vi "test - MessageReponseNoError.vi"(8 "error in (no error)":errorcluster, 11 "TestCase in":refnum<class "testcase-SyncMessage.lvclass">) -> (0 "error out":errorcluster, 3 "TestCase out":refnum<class "testcase-SyncMessage.lvclass">)   [LabVIEW 2017, in "testcase-SyncMessage.lvclass"]
uses:
  testcase-SyncMessage.lvclass
  5ae9339b-24d8-490e-a9d6-72eb2a7b92ce.vi
  <vilib>/addons/_JKI Toolkits/VI Tester/TestCase.llb/TestCase.lvclass
  src/user.lib/_NEVSTOP/Communicable State Machine(CSM)/Communicable State Machine.lvlib
  C:/Program Files (x86)/National Instruments/LabVIEW 2017/vi.lib/addons/_JKI Toolkits/VI Tester/TestCase.llb/TestCase.lvclass
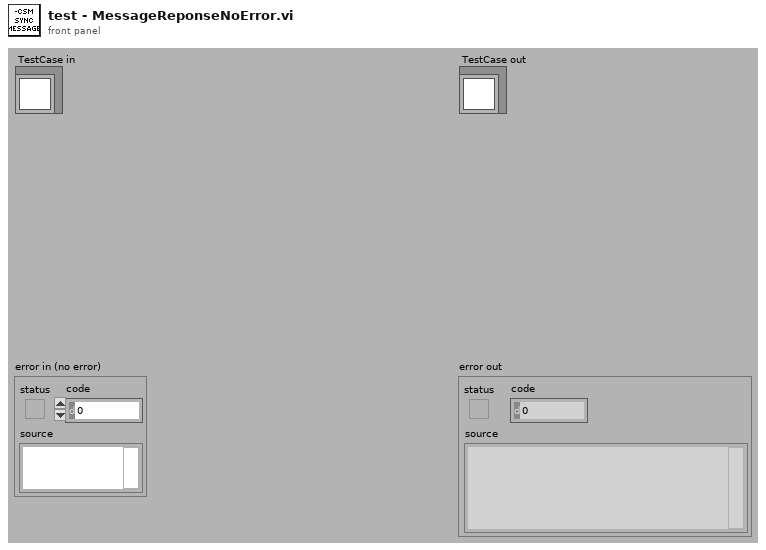
[diagram p1: front panel]
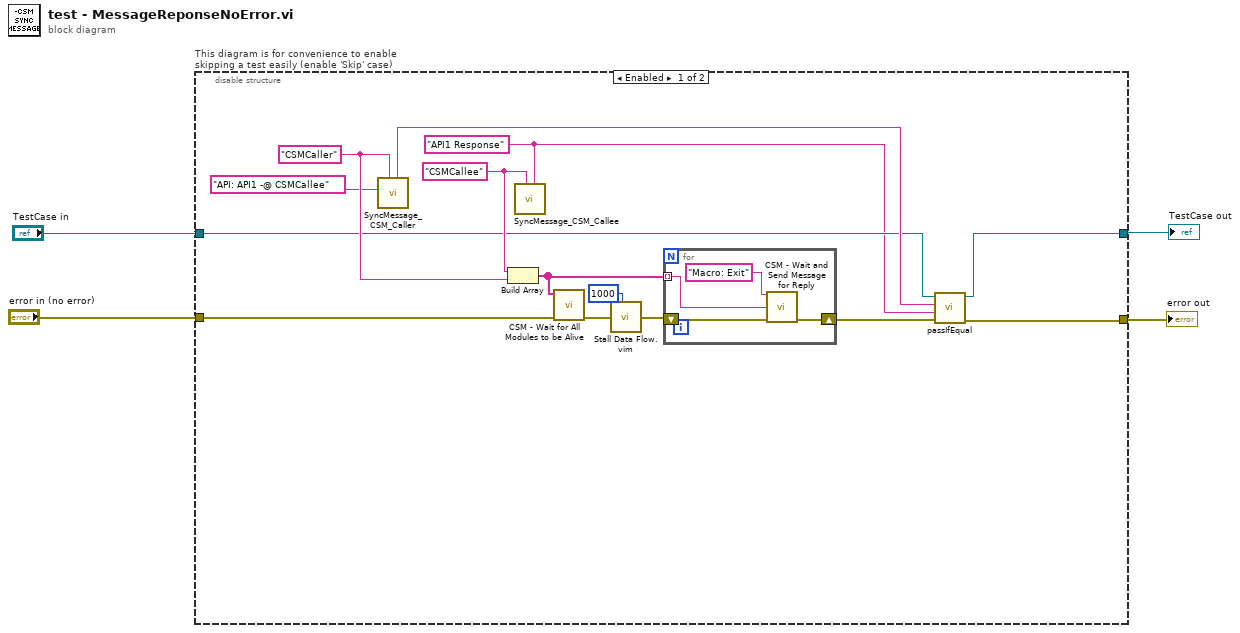
[diagram p0: block diagram]
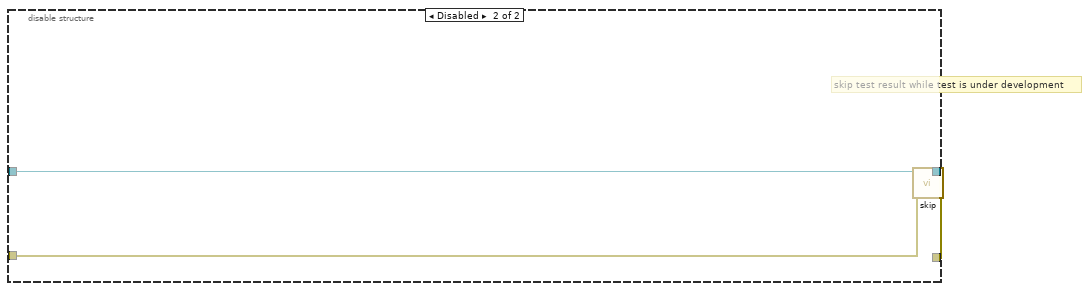
[diagram p2: hidden frame]
diagram:
  n1 = disable-structure "This diagram is for convenience to enable skipping a test easily (enable 'Skip' case)" shown="Enabled" {
    disable-tunnel: "TestCase in" -> [w7 w26]
    disable-tunnel: [w8 w24] -> w2
    disable-tunnel: [w9 w25] -> w1
    disable-tunnel: "error in (no error)" -> [w18 w23]
    frame Enabled {
      w6 = "API1 Response" ("API response in")
      w16 = "CSMCallee" ("Name (\"\" to Use UUID)")
      w17 = "CSMCaller" ("Name (\"\" to Use UUID)")
      n2 = call "SyncMessage_CSM_Caller.vi"("Name (\"\" to Use UUID)"=w17, "Intermodule Message in"="API: API1 -@ CSMCallee") -> ("API Response out"=w15:string)  [unwired: 9 in]
      n3 = Build Array(w16, w17) -> (w14:string[])
      n4 = call "SyncMessage_CSM_Callee.vi"("API response in"=w6, "Name (\"\" to Use UUID)"=w16) -> ()  [unwired: 10 in]
      n5 = call "CSM - Wait for All Modules to be Alive.vi"("Error In"=w18, "CSM Names"=w14) -> ("error out"=w13:errorcluster)  [unwired: 7 in, 2 out]
      n6 = call "Stall Data Flow.vim"("value in"=w13, "milliseconds to wait"=u32 1000) -> ("value out"=w12:errorcluster)  [unwired: 1 out]
      n7 = for {
        shift-right: [w20] -> w10
        shift-left: w12 -> [w21]
        tunnel: w14 -> [w19] mode=indexing
        n8 = call "CSM - Wait and Send Message for Reply.vi"("State"="Macro: Exit", "Target Module"=w19, "Error In (No Error)"=w21) -> ("error out"=w20:errorcluster)  [unwired: 10 in, 2 out]
      }
      n9 = call-dynamic "passIfEqual.vi"("error in (no error)"=w10, "y"=w6, "x"=w15, "TestCase in"=w7) -> ("error out"=w9:errorcluster, "TestCase out"=w8:refnum<class "testcase-SyncMessage.lvclass">)  [unwired: 6 in]
    }
    frame Disabled {
      # "skip test result while test is under development"
      n10 = call <vilib>:"skip.vi"("error in (no error)"=w23, "TestCase in"=w26) -> ("error out"=w25:errorcluster, "TestCase out"=w24:refnum<class "testcase-SyncMessage.lvclass">)  [unwired: 8 in]
    }
  }
  "error out" <- w1
  "TestCase out" <- w2
